vi "Reduce Speed.vi"(1 "Reduction Factor":dbl=2.0 format="%#_13g", 2 "Drive Controls":T1) -> (0 "Drive Controls":T1)   [LabVIEW 2014]
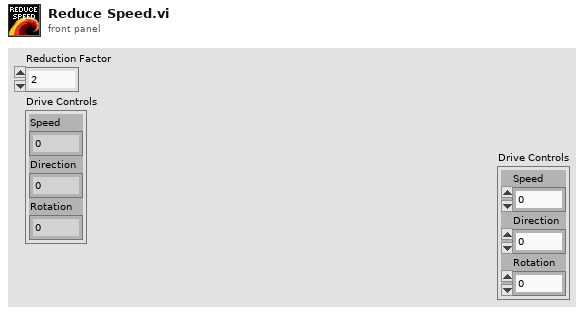
[diagram p1: front panel]
types:
  T1 = cluster{"Speed":dbl, "Direction":dbl, "Rotation":dbl}
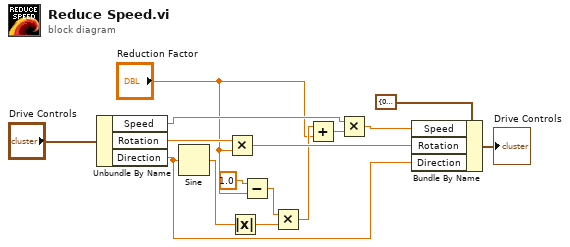
[diagram p0: block diagram]
diagram:
  n1 = Unbundle By Name("Drive Controls") -> ("Speed"=w14:dbl, "Rotation"=w13:dbl, "Direction"=w2:dbl)
  n2 = Sine(x=w2) -> (sin(x)=w4:dbl)
  n3 = Multiply(x=w13, y="Reduction Factor") -> (x*y=w10:dbl)
  n4 = Absolute Value(x=w4) -> (abs(x)=w3:dbl)
  n5 = Subtract(x=1.0, y="Reduction Factor") -> (x-y=w7:dbl)
  n6 = Multiply(x=w7, y=w3) -> (x*y=w6:dbl)
  n7 = Add(x=w6, y="Reduction Factor") -> (x+y=w1:dbl)
  n8 = Multiply(x=w14, y=w1) -> (x*y=w11:dbl)
  n9 = Bundle By Name(cluster=T1 {"Speed"=0.0, "Direction"=0.0, "Rotation"=0.0} ("Drive Controls 2"), "Speed"=w11, "Rotation"=w10, "Direction"=w2) -> (→"Drive Controls":T1)
